vi "Gerar sinal para ligar um LED.vi"() -> ()   [LabVIEW 2020]
panel:
  in  "stop":bool
  out "LED":bool
  in  "Interruptor":bool
  # "Controle de LED através do LABVIEW"
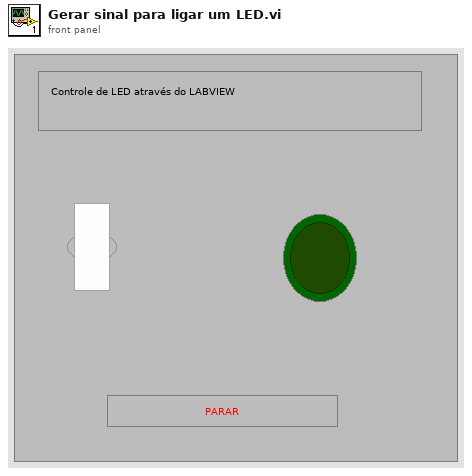
[diagram p1: front panel]
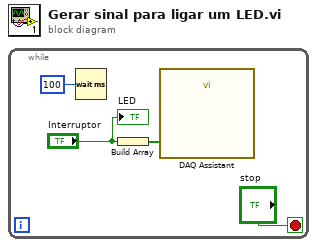
[diagram p0: block diagram]
diagram:
  n1 = while {
    stop <- "stop" stop-if-true
    n2 = Wait (ms)(milliseconds to wait=u32 100) -> ()  [unwired: 1 out]
    n3 = Build Array("Interruptor") -> (w2:bool[])
    n4 = call "DAQ Assistant"("data"=w2) -> ()  [unwired: 17 in, 2 out]
    "LED" <- "Interruptor"
  }
